vi "Example 2.vi"() -> ()   [LabVIEW 2016]
panel:
  out "length":i32
  out "String":string
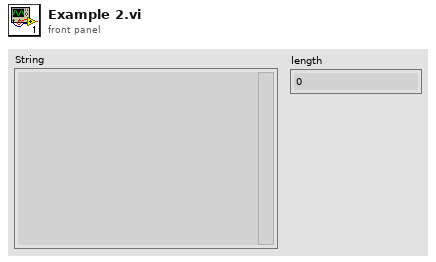
[diagram p1: front panel]
types:
  T1 = typedef "Com_Matrix220_Buffer Data.ctl" = cluster{"Connection ID":refnum<k5>}
  T2 = enum16{"Standard", "Buffered", "CRLF", "Immediate"}
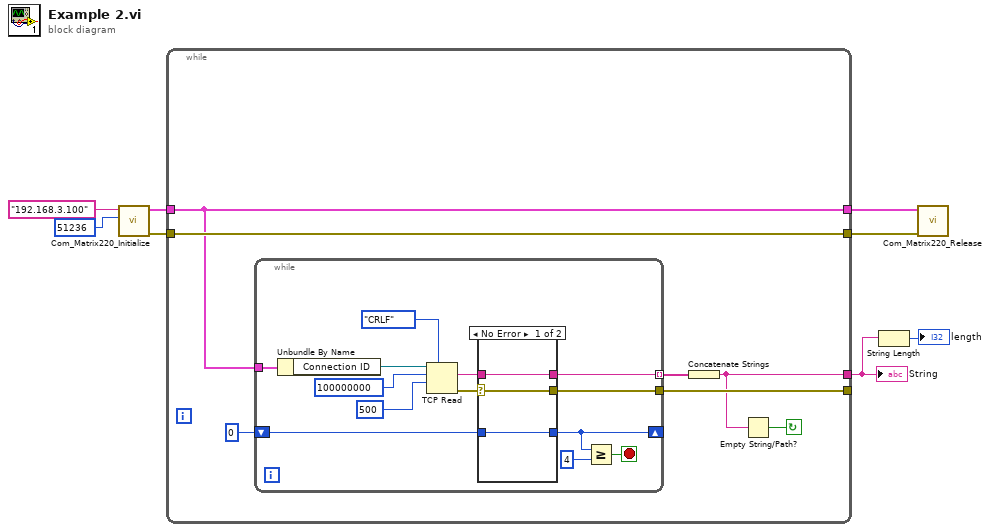
[diagram p0: block diagram]
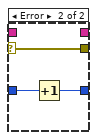
[diagram p2: hidden frame]
diagram:
  n1 = call "Com_Matrix220_Initialize.vi"("Remote Port"=u16 51236, "IP Address"="192.168.3.100") -> ("error out"=w5:errorcluster, "Buffer Data"=w6:T1)  [unwired: 8 in]
  n2 = while {
    tunnel: w6 -> [w14]
    tunnel: w5 -> [w15]
    tunnel: [w14] -> w4
    tunnel: [w15] -> w3
    tunnel: [w11] -> _
    tunnel: [w9] -> w2
    stop <- w10 continue-if-true
    n3 = while {
      tunnel: w14 -> [w28]
      shift-right: [w18] -> _
      shift-left: 0 -> [w19]
      tunnel: [w21] -> w11
      tunnel: [w20] -> w12 mode=indexing
      stop <- w16 stop-if-true
      n4 = Unbundle By Name(w28) -> ("Connection ID"=w27:refnum<k5>)
      n5 = TCP Read(connection ID=w27, bytes to read=100000000, 7:T2."CRLF" ("mode (standard)"), 9:500 ("timeout ms (25000)")) -> (data out=w22:string, error out=w23:errorcluster)  [unwired: 1 in, 1 out]
      n6 = case shown="No Error" w23 {
        selector: w23 -> [w31 w34]
        tunnel: w22 -> [w30 _]
        tunnel: [w31 w34] -> w21
        tunnel: [w30 _] -> w20
        tunnel: w19 -> [w29 w33]
        tunnel: [w29 w32] -> w18
        frame No Error {
        }
        frame Error {
          n7 = Increment(x=w33) -> (x+1=w32:i32)
        }
      }
      n8 = Greater Or Equal?(x=w18, y=4) -> (x >= y?=w16:bool)
    }
    n9 = Concatenate Strings(w12) -> (w9:string)
    n10 = Empty String/Path?(string/path=w9) -> (empty?=w10:bool)
  }
  "String" <- w2
  n11 = String Length(string=w2) -> (length=→"length":i32)
  n12 = call "Com_Matrix220_Release.vi"("error in"=w3, "Buffer Data"=w4) -> ()  [unwired: 9 in, 1 out]
